vi "Parameters from Front Panel.vi"(8 "error in (no error)":errorcluster, 11 "Menu object array in":refnum<class "Menu object array.lvclass">) -> (0 "error out":errorcluster, 3 "Menu object array out":refnum<class "Menu object array.lvclass">)   [LabVIEW 2015, in "Menu object array.lvclass"]
uses:
  Menu object array.lvclass
  Controls/Menu object array.ctl
  Controls/Menu object.ctl
  Menu object parameters.lvclass
  Menu object array.lvclass/Menu object array.ctl
  Menu object parameters.lvclass/Menu object parameters.ctl
  Mag Lab Measure Interface/Mag Lab Measure UI.lvclass
  Mag Lab Error Handler/Mag Lab Error Handler.lvclass
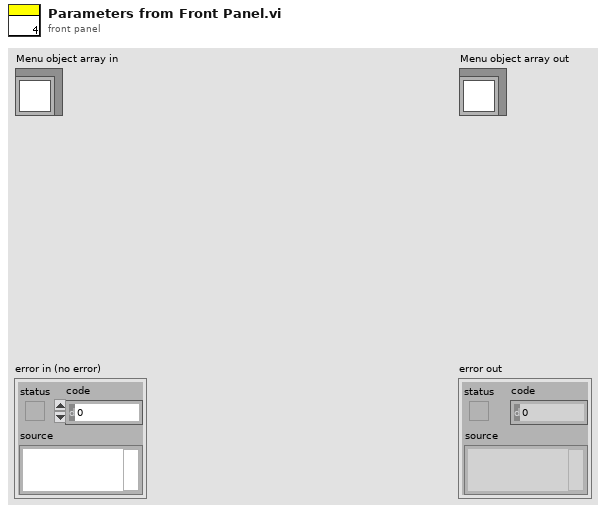
[diagram p1: front panel]
types:
  T1 = typedef "Menu object array.ctl" = T2[]
  T2 = typedef "Menu object.ctl" = cluster{"Object name":u16, "Open parameters":bool, "Remove Button":bool}
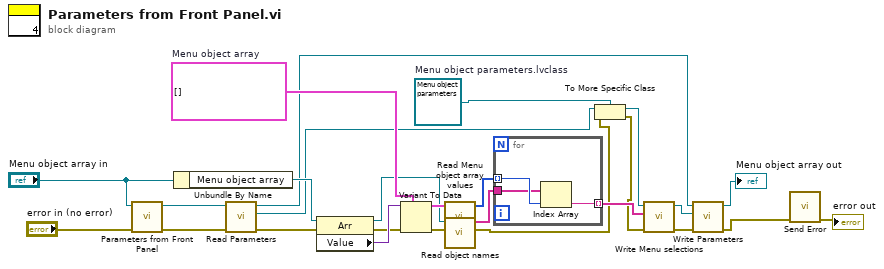
[diagram p0: block diagram]
diagram:
  w15 = refnum<class "Menu object parameters.lvclass"> refnum  # Menu object parameters.lvclass
  w24 = T1 []  # Menu object array
  n1 = call-parent "Parameters from Front Panel.vi"("error in (no error)"="error in (no error)", "Mag Lab Measure Interface in"="Menu object array in") -> ("error out"=w9:errorcluster, "Mag Lab Measure Interface out"=w10:refnum<class "Menu object array.lvclass">)  [unwired: 8 in]
  n2 = Unbundle By Name("Menu object array in") -> ("Menu object array"=w26:refnum<vi>)
  n3 = call-dynamic "Read Parameters.vi"("error in (no error)"=w9, "Mag Lab Root in"=w10) -> ("error out"=w14:errorcluster, "Mag Lab Parameters.lvclass"=w13:refnum<class "Mag Lab Parameters.lvclass">, "Mag Lab Root out"=w6:refnum<class "Menu object array.lvclass">)  [unwired: 7 in]
  n4 = property class="Arr"(reference=w26, error in=w14) -> (reference out=w20:refnum<vi>, error out=w22:errorcluster, "Value"=w25:variant)
  n5 = Variant To Data(error in=w22, type=w24, Variant=w25) -> (data=w23:T1, error out=w19:errorcluster)
  n6 = call "Read Menu object array values.vi"("Menu object array"=w23) -> ("Values"=w21:u16[])  [unwired: 6 in, 4 out]
  n7 = call "Read object names.vi"("Error In"=w19, "Menu object array ref"=w20) -> ("Error Out"=w4:errorcluster, "Object names"=w18:string[])  [unwired: 8 in]
  n8 = for {
    tunnel: w21 -> [w29] mode=indexing
    tunnel: w18 -> [w28]
    tunnel: [w27] -> w17 mode=indexing
    n9 = Index Array(array=w28, index=w29) -> (element=w27:string)
  }
  n10 = To More Specific Class(target class=w15, reference=w13, error in=w4) -> (specific class reference=w16:refnum<class "Menu object parameters.lvclass">, error out=w3:errorcluster)
  n11 = call "Write Menu selections.vi"("error in (no error)"=w3, "Menu selections"=w17, "Menu object parameters in"=w16) -> ("error out"=w8:errorcluster, "Menu object parameters out"=w7:refnum<class "Menu object parameters.lvclass">)  [unwired: 7 in]
  n12 = call-dynamic "Write Parameters.vi"("error in (no error)"=w8, "Mag Lab Parameters.lvclass"=w7, "Menu object array in"=w6) -> ("error out"=w2:errorcluster, "Menu object array out"=→"Menu object array out":refnum<class "Menu object array.lvclass">)  [unwired: 7 in]
  n13 = call "Send Error.vi"("error in (no error)"=w2) -> ("error out"=→"error out":errorcluster)  [unwired: 9 in, 1 out]
